vi "mat2pos.vi"(11 "Real Matrix":T1) -> (3 "pos":dbl[](array[numeric]))   [LabVIEW 2012]
uses:
  <vilib>/Analysis/Matrix/Datatypes/RealMatrix.ctl
  <vilib>/Analysis/Matrix/NI_Matrix.lvlib
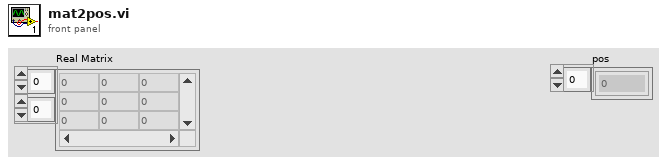
[diagram p1: front panel]
types:
  T1 = typedef "NI_Matrix.lvlib/RealMatrix.ctl" = dbl[][]
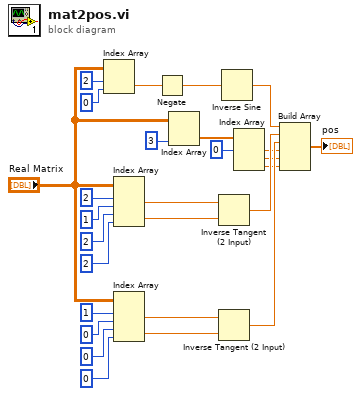
[diagram p0: block diagram]
diagram:
  n1 = Index Array(array="Real Matrix", index (row)=2, index (col)=0 ("disabled index (col)")) -> (element=w25:dbl)
  n2 = Index Array(array="Real Matrix", index (row) #1=2 ("index (row)"), index (col) #1=1 ("disabled index (col)"), index (row) #2=2 ("index (row)"), index (col) #2=2 ("index (row)")) -> (element #1=w19:dbl, element #2=w18:dbl)
  n3 = Index Array(array="Real Matrix", index (row) #1=1 ("index (row)"), index (col) #1=0 ("disabled index (col)"), index (row) #2=0 ("index (row)"), index (col) #2=0 ("index (row)")) -> (element #1=w16:dbl, element #2=w17:dbl)
  n4 = Negate(x=w25) -> (-x=w24:dbl)
  n5 = Index Array(array="Real Matrix", index (col)=3 ("disabled index (col)")) -> (element=w10:dbl[])  [unwired: 1 in]
  n6 = Inverse Tangent (2 Input)(1:w18, 2:w19) -> (0:w7:dbl)
  n7 = Inverse Tangent (2 Input)(1:w17, 2:w16) -> (0:w6:dbl)
  n8 = Inverse Sine(1:w24) -> (0:w8:dbl)
  n9 = Index Array(array=w10, index #1=0 ("index")) -> (element #1=w5:dbl, element #2=w4:dbl, element #3=w3:dbl)  [unwired: 2 in]
  n10 = Build Array(w8, w7, w6, w5, w4, w3) -> (→"pos":dbl[])
